vi "Configure AM Internal [AM].vi"(7 "modulation waveform (Sine)":i32(ring)=1 items=["Sine"=1, "Square"=2, "Triangle"=3, "Ramp Up"=4, "Ramp Down"=5], 8 "error in (no error)":errorcluster, 9 "modulation frequency (1000 Hz)":dbl[unit]=1000.0 format="%^.2e", 10 "modulation depth (0.00 %)":dbl format="%.3f", 11 "CS++Fgen in":refnum<class "CS++Fgen.lvclass">) -> (0 "error out":errorcluster, 3 "CS++Fgen out":refnum<class "CS++Fgen.lvclass">)   [LabVIEW 2013, in "CS++Fgen.lvlib" / "CS++Fgen.lvclass"]
doc: "This VI configures the properties that control the function generator's internal amplitude modulation source. These properties are the modulation depth, waveform, and frequency.\n\nNotes:\n\n(1) This VI is part of the IviFgenModulateAM [AM] extension group."
uses:
  CS++Fgen.lvclass
  Core/Classes/CS++ProcessVariables/ProcessVariable/PV.lvclass
  CS++Fgen.lvclass/CS++Fgen.ctl
  Core/Classes/CS++ProcessVariables/PVConnection/PVConnection.lvclass
  Core/Classes/CS++ProcessVariables/ProcessVariable/PV.lvclass/PV.ctl
  Core/Classes/CS++ProcessVariables/ProcessVariable/Write Data.vi
  Core/Classes/CS++ProcessVariables/ProcessVariable/Write Timestamp.vi
  Core/Classes/CS++ProcessVariables/ProcessVariable/Write Quality.vi
  Core/Classes/CS++ProcessVariables/ProcessVariable/Write status.vi
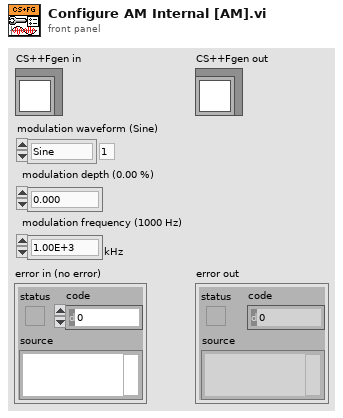
[diagram p1: front panel]
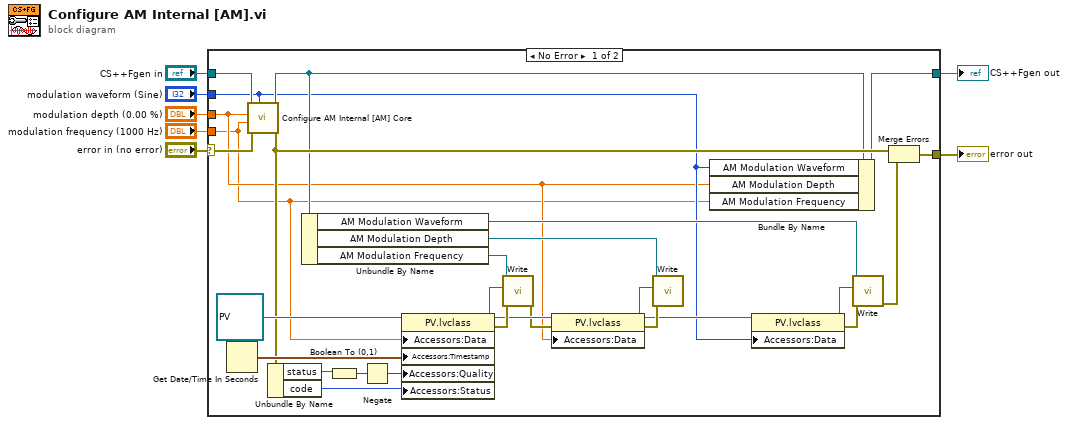
[diagram p0: block diagram]
diagram:
  n1 = case shown="No Error" "error in (no error)" {
    selector: "error in (no error)" -> [w32 w35]
    tunnel: [w12 w35] -> w6
    tunnel: [w22 w34] -> w4
    tunnel: "CS++Fgen in" -> [w33 w34]
    tunnel: "modulation waveform (Sine)" -> [w10 _]
    tunnel: "modulation depth (0.00 %)" -> [w9 _]
    tunnel: "modulation frequency (1000 Hz)" -> [w8 _]
    frame No Error {
      n2 = Get Date/Time In Seconds() -> (seconds since 1Jan1904=w31:timestamp)
      n3 = call-dynamic "Configure AM Internal [AM] Core.vi"("modulation waveform (Sine)"=w10, "error in (no error)"=w32, "modulation frequency (1000 Hz)"=w8, "modulation depth (0.00 %)"=w9, "CS++Fgen in"=w33) -> ("error out"=w24:errorcluster, "CS++Fgen out"=w23:refnum<class "CS++Fgen.lvclass">)  [unwired: 5 in]
      n4 = Unbundle By Name(w24) -> ("status"=w28:bool, "code"=w26:i32)
      n5 = Unbundle By Name(w23) -> ("AM Modulation Waveform"=w14:refnum<class "PVConnection.lvclass">, "AM Modulation Depth"=w19:refnum<class "PVConnection.lvclass">, "AM Modulation Frequency"=w21:refnum<class "PVConnection.lvclass">)
      n6 = Boolean To (0,1)(Boolean=w28) -> (0, 1=w27:i16)
      n7 = Negate(x=w27) -> (-x=w25:i16)
      n8 = property class="PV.lvclass"(reference=refnum<class "PV.lvclass"> refnum ("PV"), "Accessors:Data"=w8, "Accessors:Timestamp"=w31, "Accessors:Quality"=w25, "Accessors:Status"=w26) -> (reference out=w18:refnum<class "PV.lvclass">, error out=w29:errorcluster)  [unwired: 1 in]
      n9 = call-dynamic "Write.vi"("error in (no error)"=w29, "PV"=w18, "PVConnection in"=w21) -> ("error out"=w17:errorcluster)  [unwired: 7 in, 1 out]
      n10 = property class="PV.lvclass"(reference=w18, error in=w17, "Accessors:Data"=w9) -> (reference out=w13:refnum<class "PV.lvclass">, error out=w20:errorcluster)
      n11 = call-dynamic "Write.vi"("error in (no error)"=w20, "PV"=w13, "PVConnection in"=w19) -> ()  [unwired: 7 in, 2 out]
      n12 = Bundle By Name(cluster=w23, "AM Modulation Waveform"=w10, "AM Modulation Depth"=w9, "AM Modulation Frequency"=w8) -> (w22:refnum<class "CS++Fgen.lvclass">)
      n13 = property class="PV.lvclass"(reference=w13, "Accessors:Data"=w10) -> (reference out=w15:refnum<class "PV.lvclass">, error out=w16:errorcluster)  [unwired: 1 in]
      n14 = call-dynamic "Write.vi"("error in (no error)"=w16, "PV"=w15, "PVConnection in"=w14) -> ("error out"=w11:errorcluster)  [unwired: 7 in, 1 out]
      n15 = Merge Errors(w24, w11) -> (w12:errorcluster)
    }
    frame Error {
    }
  }
  "error out" <- w6
  "CS++Fgen out" <- w4
